vi "Exercise1.1-Adder.vi"() -> ()   [LabVIEW 2013]
panel:
  out "a+b":dbl
  in  "b":dbl
  in  "a":dbl
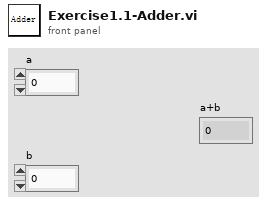
[diagram p1: front panel]
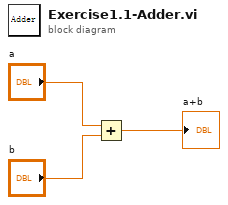
[diagram p0: block diagram]
diagram:
  n1 = Add(x="a", y="b") -> (x+y=→"a+b":dbl)
